vi "obj_DataLog Aggregate New Points.vi"(0 "method":T1, 9 "tag index in":i32) -> (10 "tag index out":i32)   [LabVIEW 2012]
doc: "This object aggregates the newly buffered points. This causes the points to be copied from the tag buffer to the aggregation buffer in a manner that is dependent on the selected logging algorithm and its parameterisation.\n\nThis object is called periodically by the aggregator plug-in. It is also called when a tag of the live database is being queried so as to move all available data over to the aggregation buffer for flush preceding the retrieval. This object is protected such that {aggregate} calls before {initialize} or after {cleanup} are inert."
uses:
  typedefs/t_DataLog Aggregate New Points Methods.ctl
  typedefs/clusters/t_DataLog Point.ctl
  typedefs/t_DataLog Tag Buffers Methods.ctl
  typedefs/t_DataLog Tag Info List Methods.ctl
  typedefs/t_DataLog Aggregation Buffer Methods.ctl
  subvis/private/glb_DataLog Runtime Parameterisation.vi
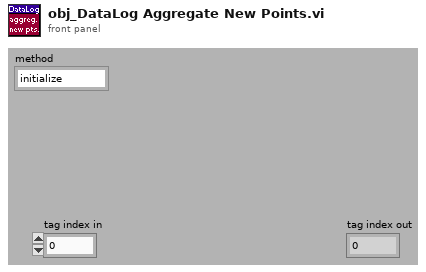
[diagram p1: front panel]
types:
  T1 = typedef "t_DataLog Aggregate New Points Methods.ctl" = enum16{"initialize", "aggregate", "cleanup"}
  T2 = typedef "t_DataLog Point.ctl" = cluster{"time":dbl, "value":dbl}
  T3 = typedef "t_DataLog Tag Buffers Methods.ctl" = enum16{"initialize", "inert", "write", "read", "read oldest", "read last", "cleanup"}
  T4 = typedef "t_DataLog Tag Info List Methods.ctl" = enum16{"initialize", "create", "create empty", "rename", "delete", "test tag", "get", "get by name", "get default", "get list", "get path", "get subsets", "set subsets", "set config", "set capacity", "#tags", "go live", "set unlocked", "set mirrored"}
  T5 = typedef "t_DataLog Aggregation Buffer Methods.ctl" = enum16{"initialize", "write", "write special", "flush", "flush next", "flush next if", "setup recovery", "update recovery", "verify recovery", "dummy flush ", "cleanup"}
  T6 = typedef "t_DataLog Tag Config.ctl" = cluster{"name":string, "unit":string, "temporal":T7, "value":T8, "index":i32, "capacity":i32, "is meta?":bool, "mincapacity":i32, "deadband":dbl, "limit delay":dbl, "format":T9, "precision":u8, "undefine":bool, "update":bool, "update period":u16, "expression":string, "description":string, "logging algorithm":T10, "logging parameters":dbl[]}
  T7 = typedef "t_DataLog Temporal Types.ctl" = enum16{"set&hold", "sample", "event"}
  T8 = typedef "t_DataLog Value Types.ctl" = enum16{"number", "string"}
  T9 = typedef "t_DataLog Numerical Format.ctl" = enum8{"fractional", "exponential", "engineering"}
  T10 = typedef "t_DataLog Logging Algorithms.ctl" = enum16{"nothing", "changes", "everything", "every Nth", "time threshold", "value threshold + prior", "t or v threshold", "t or v threshold + prior"}
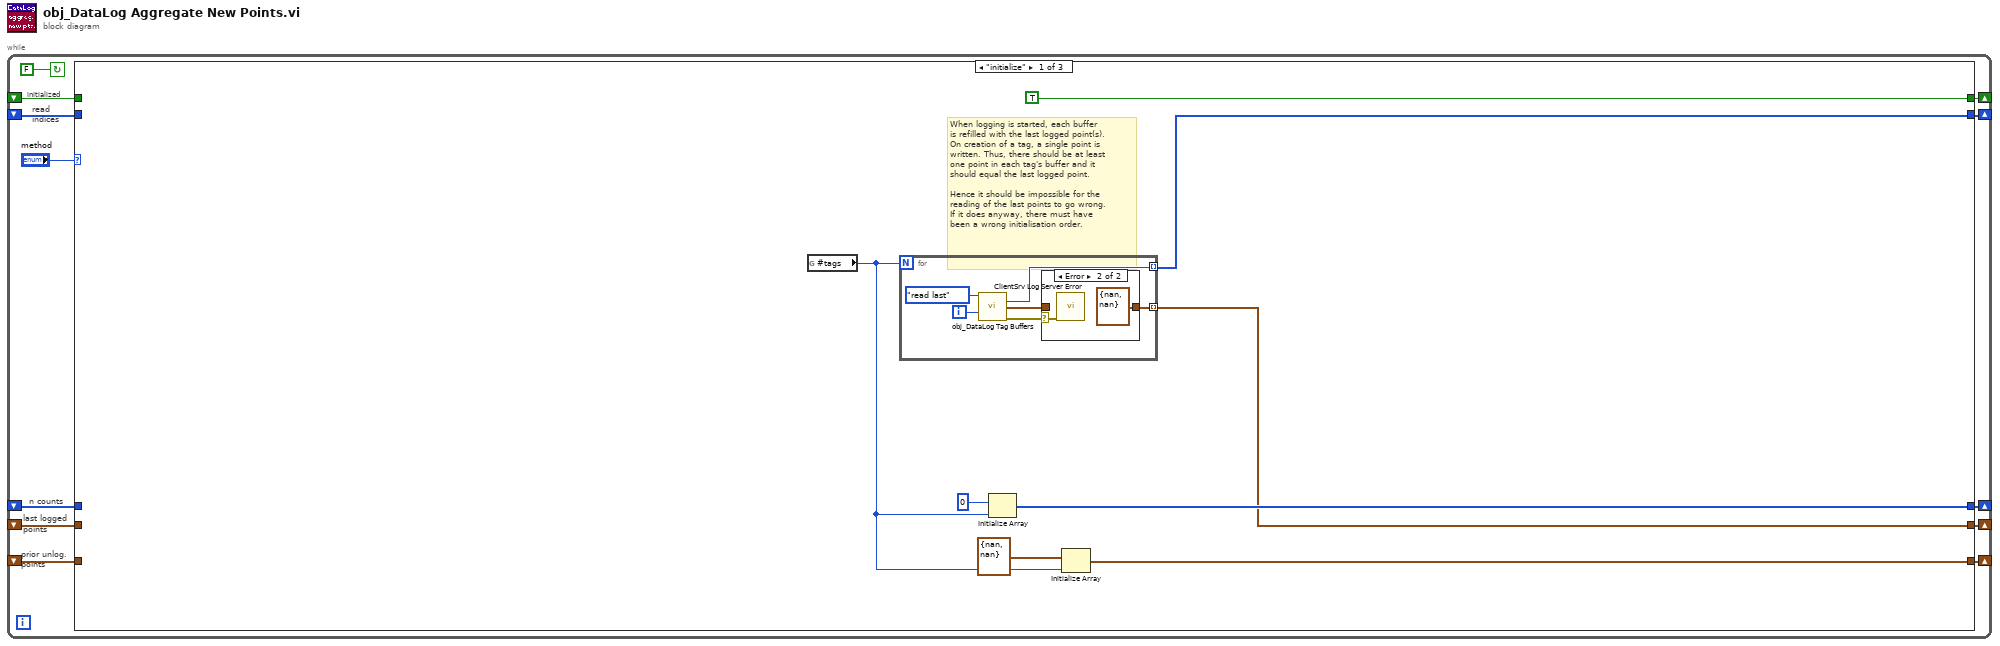
[diagram p0: block diagram]
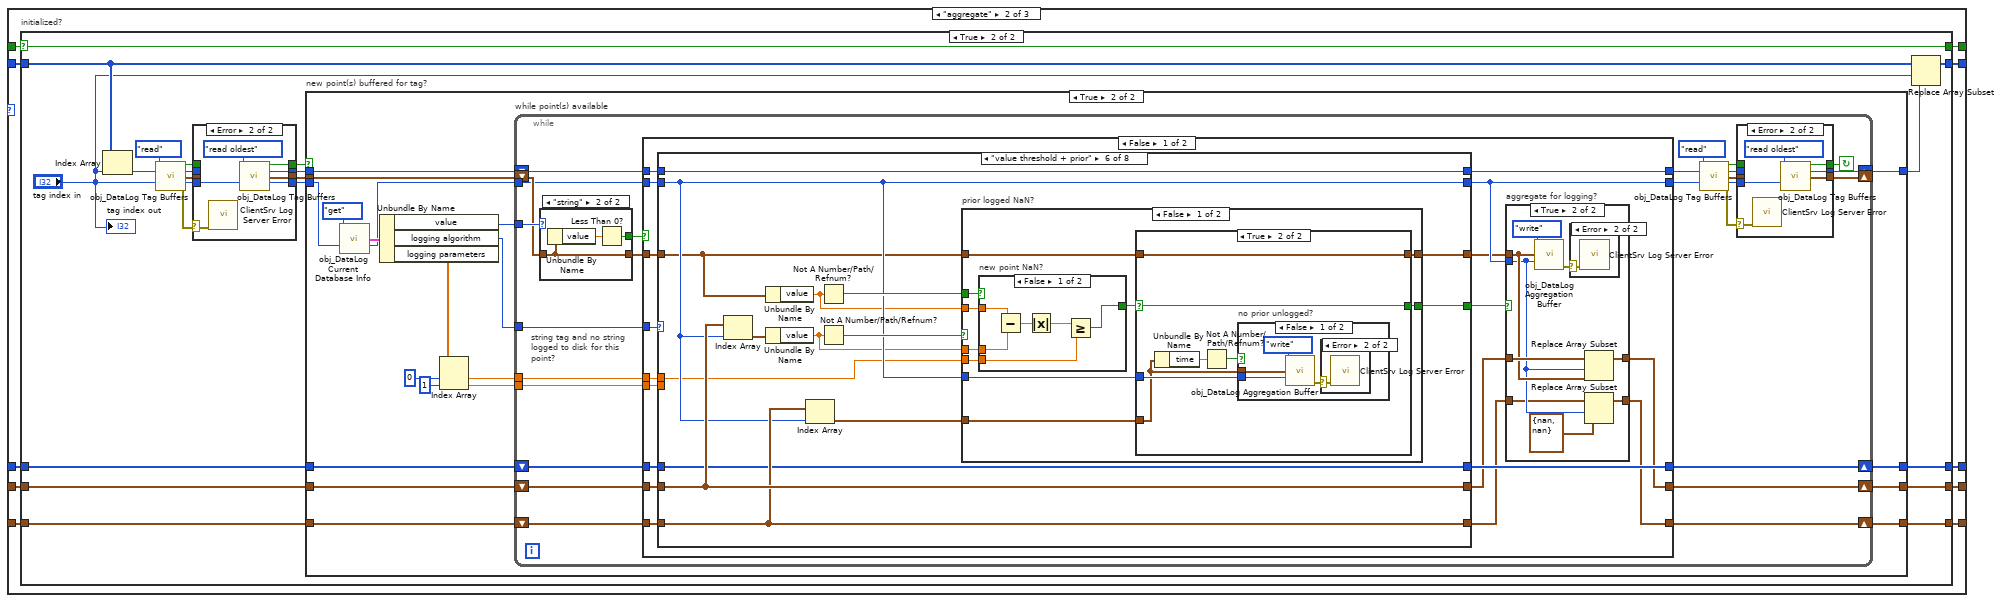
[diagram p3: hidden frame]
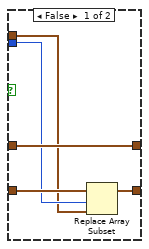
[diagram p8: hidden frame]
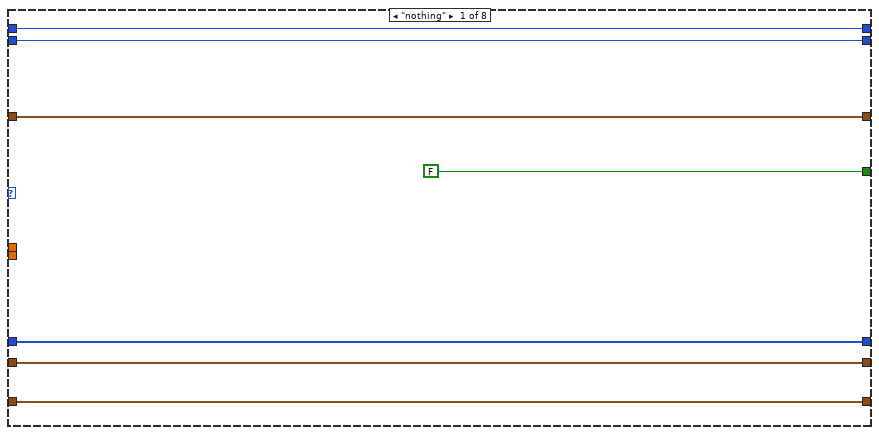
[diagram p10: hidden frame]
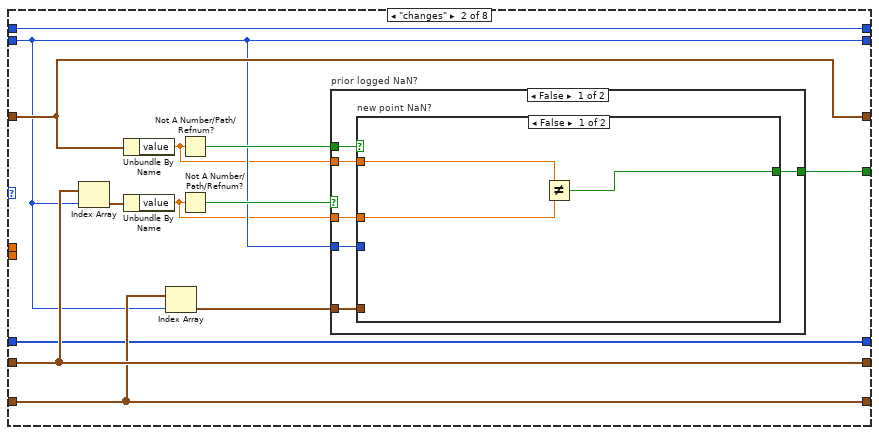
[diagram p11: hidden frame]
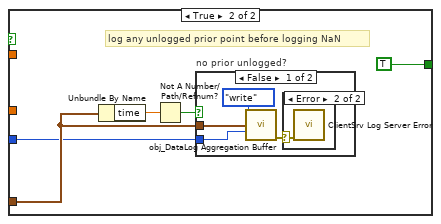
[diagram p12: hidden frame]
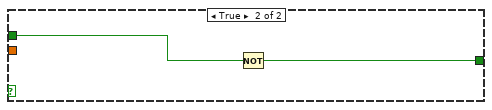
[diagram p15: hidden frame]
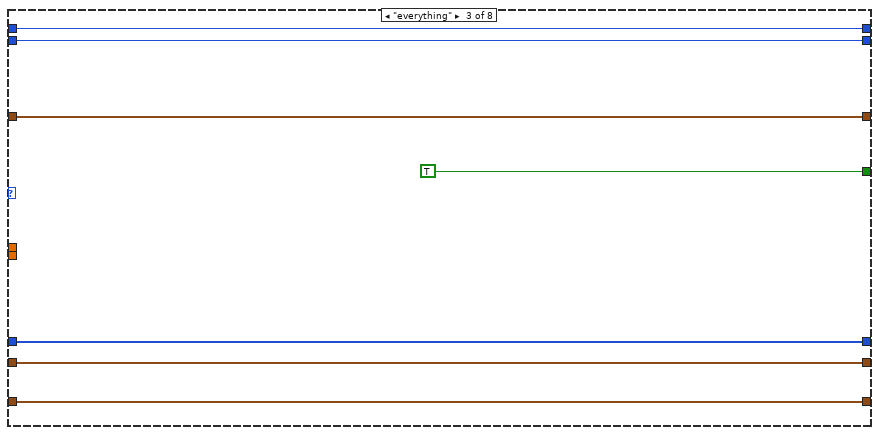
[diagram p16: hidden frame]
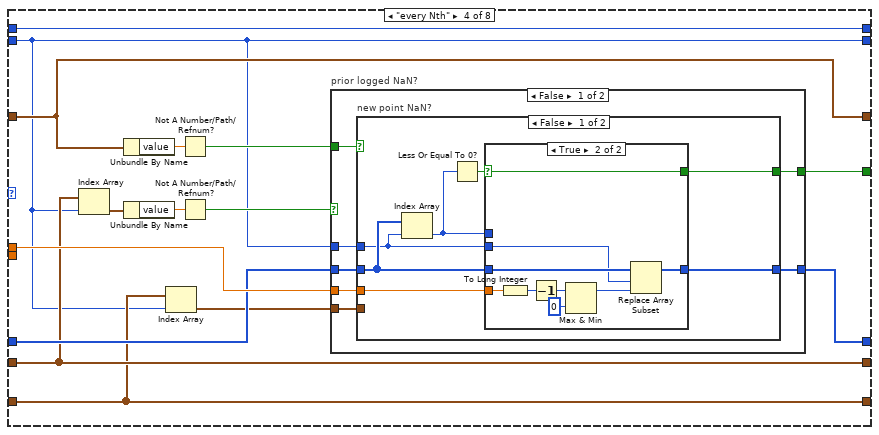
[diagram p17: hidden frame]
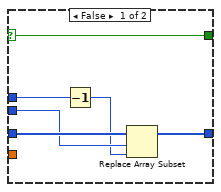
[diagram p18: hidden frame]
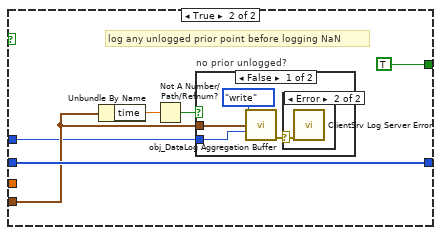
[diagram p19: hidden frame]
diagram:
  n1 = while {
    shift-right: [w9] -> _
    shift-left: _ -> [w10]
    shift-right: [w8] -> _
    shift-left: _ -> [w7]
    shift-right: [w6] -> _
    shift-left: _ -> [w5]
    shift-right: [w4] -> _
    shift-left: _ -> [w3]
    shift-right: [w2] -> _
    shift-left: _ -> [w1]
    stop <- FALSE continue-if-true
    # "prior unlog.\npoints"
    # "last logged\npoints"
    # "n counts"
    # "initialized"
    # "read\nindices"
    n2 = case shown="\"initialize\"" "method" {
      tunnel: w10 -> [_ w39 w520]
      tunnel: [w20 w38 w519] -> w9
      tunnel: [TRUE w36 FALSE] -> w8
      tunnel: w7 -> [_ w37 _]
      tunnel: [w17 w34 w515] -> w6
      tunnel: w5 -> [_ w35 w516]
      tunnel: [w13 w32 w512] -> w4
      tunnel: w3 -> [_ w33 w511]
      tunnel: [w15 w31 w508] -> w2
      tunnel: w1 -> [_ w30 w509]
      frame "initialize" {
        # "When logging is started, each buffer\nis refilled with the last logged point(s).\nOn creation of a tag, a single point is\nwritten. Thus, there should be at least\none point in each tag's buffer and it\nshould equal the last logged point.\n\nHence it should be impossible for the\nreading of the last points to go wrong.\nIf it does anyway, there must have\nbeen a wrong initialisation order."
        n3 = global read "glb_DataLog Runtime Parameterisation.vi" "#tags"() -> (w14:i32)
        n4 = for {
          N: w14 -> [_]
          tunnel: [w24] -> w20 mode=indexing
          tunnel: [w21] -> w13 mode=indexing
          i -> [w25]
          n5 = call "obj_DataLog Tag Buffers.vi"("method"=t_DataLog_Tag_Buffers_Methods."read last", "tag index"=w25) -> ("read index out"=w24:i32, "point out"=w22:T2, "error out"=w23:errorcluster)  [unwired: 9 in, 2 out]
          n6 = case shown="Error" w23 {
            selector: w23 -> [_ w29]
            tunnel: w22 -> [w27 _]
            tunnel: [w27 T2 {"time"=nan, "value"=nan} ("point")] -> w21
            frame No Error {
            }
            frame Error {
              n7 = call "ClientSrv Log Server Error.vi"("error (use message)"=w29) -> ()  [unwired: 15 in]
            }
          }
        }
        n8 = Initialize Array(0, w14) -> (w17:i32[])
        n9 = Initialize Array(T2 {"time"=nan, "value"=nan} ("point"), w14) -> (w15:T2[])
      }
      frame "aggregate" {
        n10 = case "initialized?" shown="True" w37 {
          selector: w37 -> [w44 w63]
          tunnel: w39 -> [w43 w66]
          tunnel: [w43 w65] -> w38
          tunnel: [w44 w63] -> w36
          tunnel: w35 -> [w42 w62]
          tunnel: [w42 w61] -> w34
          tunnel: [w41 w59] -> w32
          tunnel: w33 -> [w41 w60]
          tunnel: [w40 w58] -> w31
          tunnel: w30 -> [w40 w57]
          frame False {
            # "protects against on-query flush calls when aggregation is inactive"
          }
          frame True {
            n11 = Index Array(array=w66, index="tag index in") -> (element=w50:i32)
            n12 = call "obj_DataLog Tag Buffers.vi"("method"=t_DataLog_Tag_Buffers_Methods."read", "read index in"=w50, "tag index"="tag index in") -> ("available?"=w53:bool, "read index out"=w51:i32, "point out"=w55:T2, "tag index dup"=w54:i32, "error out"=w52:errorcluster)  [unwired: 8 in]
            n13 = case shown="Error" w52 {
              selector: w52 -> [_ w501]
              tunnel: w55 -> [w498 _]
              tunnel: w54 -> [w497 w503]
              tunnel: w53 -> [w499 _]
              tunnel: [w500 w506] -> w48
              tunnel: w51 -> [w500 _]
              tunnel: [w499 w505] -> w47
              tunnel: [w498 w504] -> w49
              tunnel: [w497 w502] -> w45
              frame No Error {
              }
              frame Error {
                n14 = call "ClientSrv Log Server Error.vi"("error (use message)"=w501) -> ()  [unwired: 15 in]
                n15 = call "obj_DataLog Tag Buffers.vi"("method"=t_DataLog_Tag_Buffers_Methods."read oldest", "tag index"=w503) -> ("available?"=w505:bool, "read index out"=w506:i32, "point out"=w504:T2, "tag index dup"=w502:i32)  [unwired: 9 in, 1 out]
              }
            }
            n16 = case "new point(s) buffered for tag?" shown="True" w47 {
              tunnel: [w70 w90] -> w64
              tunnel: w62 -> [w69 w89]
              tunnel: [w69 w88] -> w61
              tunnel: w60 -> [w68 w87]
              tunnel: [w68 w86] -> w59
              tunnel: [w67 w85] -> w58
              tunnel: w57 -> [w67 w84]
              tunnel: w49 -> [_ w83]
              tunnel: w48 -> [w70 w82]
              tunnel: w45 -> [_ w80]
              frame False {
              }
              frame True {
                n17 = call "obj_DataLog Current Database Info.vi"("method"=t_DataLog_Tag_Info_List_Methods."get", "tag index/change#"=w80) -> ("tag config out"=w79:T6, "dup tag index"=w71:i32)  [unwired: 7 in, 5 out]
                n18 = Unbundle By Name(w79) -> ("value"=w72:T8, "logging algorithm"=w75:T10, "logging parameters"=w76:dbl[])
                n19 = Index Array(array=w76, index #1=0 ("index"), index #2=1 ("index")) -> (element #1=w74:dbl, element #2=w73:dbl)
                n20 = while "while point(s) available" {
                  shift-right: [w96] -> w90
                  shift-left: w82 -> [w110]
                  shift-right: [w115] -> w88
                  shift-left: w89 -> [w116]
                  shift-right: [w113] -> w86
                  shift-left: w87 -> [w114]
                  shift-right: [w91] -> w85
                  shift-left: w84 -> [w92]
                  shift-right: [w95] -> _
                  shift-left: w83 -> [w105]
                  tunnel: w75 -> [w109]
                  tunnel: w74 -> [w108]
                  tunnel: w73 -> [w107]
                  tunnel: w72 -> [w106]
                  tunnel: w71 -> [w94]
                  stop <- w97 continue-if-true
                  n21 = case shown="\"string\"" w106 {
                    tunnel: w105 -> [w126 w127]
                    tunnel: [_ w128] -> w112
                    tunnel: [w126 w127] -> w111
                    frame "number" {
                    }
                    frame "string" {
                      n22 = Unbundle By Name(w127) -> ("value"=w129:dbl)
                      n23 = Less Than 0?(x=w129) -> (x < 0?=w128:bool)
                    }
                  }
                  n24 = case "string tag and no string logged to disk for this point?" shown="False" w112 {
                    tunnel: w110 -> [w147 w493]
                    tunnel: [w146 w493] -> w98
                    tunnel: w111 -> [w145 _]
                    tunnel: w109 -> [w144 _]
                    tunnel: w116 -> [w143 w496]
                    tunnel: [w142 w496] -> w115
                    tunnel: w114 -> [w141 w495]
                    tunnel: [w133 w495] -> w113
                    tunnel: w108 -> [w140 _]
                    tunnel: w107 -> [w139 _]
                    tunnel: w94 -> [w138 w494]
                    tunnel: [w136 w494] -> w93
                    tunnel: w92 -> [w137 w492]
                    tunnel: [w130 w492] -> w91
                    frame False {
                      n25 = case shown="\"value threshold + prior\"" w144 {
                        tunnel: w145 -> [w164 w176 w205 w214 w289 w324 w384 w435]
                        tunnel: w147 -> [w166 w182 w210 w223 w297 w337 w390 w441]
                        tunnel: [w166 w182 w210 w223 w297 w337 w390 w441] -> w146
                        tunnel: w143 -> [w169 w172 w209 w222 w283 w328 w378 w429]
                        tunnel: [w169 w172 w209 w225 w283 w328 w378 w429] -> w142
                        tunnel: w141 -> [w168 w180 w208 w218 w293 w335 w388 w439]
                        tunnel: [w168 w180 w208 w218 w293 w335 w388 w439] -> w135
                        tunnel: w140 -> [_ _ _ w224 w298 w325 w391 w442]
                        tunnel: w139 -> [_ _ _ _ _ _ w375 w426]
                        tunnel: w138 -> [w167 w174 w207 w212 w287 w330 w382 w433]
                        tunnel: [w167 w174 w207 w212 w287 w330 w382 w433] -> w136
                        tunnel: w137 -> [w165 w175 w206 w213 w288 w331 w383 w434]
                        tunnel: [w165 w175 w206 w213 w288 w331 w383 w434] -> w131
                        tunnel: [w164 w176 w205 w214 w289 w323 w384 w435] -> w134
                        tunnel: [FALSE w181 TRUE w221 w296 w336 w389 w440] -> w132
                        frame "nothing" {
                        }
                        frame "changes" {
                          n26 = Index Array(array=w180, index=w174) -> (element=w179:T2)
                          n27 = Unbundle By Name(w176) -> ("value"=w171:dbl)
                          n28 = Unbundle By Name(w179) -> ("value"=w170:dbl)
                          n29 = Index Array(array=w175, index=w174) -> (element=w173:T2)
                          n30 = Not A Number/Path/Refnum?(number/path/refnum=w171) -> (NaN/Path/Refnum?=w178:bool)
                          n31 = Not A Number/Path/Refnum?(number/path/refnum=w170) -> (NaN/Path/Refnum?=w177:bool)
                          n32 = case "prior logged NaN?" shown="False" w177 {
                            tunnel: [w188 w203] -> w181
                            tunnel: w174 -> [w187 _]
                            tunnel: w178 -> [w186 w202]
                            tunnel: w173 -> [w185 _]
                            tunnel: w170 -> [w184 _]
                            tunnel: w171 -> [w183 _]
                            frame False {
                              n33 = case "new point NaN?" shown="False" w186 {
                                tunnel: [w189 TRUE] -> w188
                                tunnel: w187 -> [_ w192]
                                tunnel: w185 -> [_ w193]
                                tunnel: w184 -> [w190 _]
                                tunnel: w183 -> [w191 _]
                                frame False {
                                n34 = Not Equal?(x=w191, y=w190) -> (x != y?=w189:bool)
                                }
                                frame True {
                                # "log any unlogged prior point before logging NaN"
                                n35 = Unbundle By Name(w193) -> ("time"=w195:dbl)
                                n36 = Not A Number/Path/Refnum?(number/path/refnum=w195) -> (NaN/Path/Refnum?=w194:bool)
                                n37 = case "no prior unlogged?" shown="False" w194 {
                                tunnel: w193 -> [w198 _]
                                tunnel: w192 -> [w197 _]
                                frame False {
                                n38 = call "obj_DataLog Aggregation Buffer.vi"("method"=t_DataLog_Aggregation_Buffer_Methods."write", "point"=w198, "tag index"=w197) -> ("error out"=w200:errorcluster)  [unwired: 11 in, 1 out]
                                n39 = case shown="Error" w200 {
                                selector: w200 -> [_ w201]
                                frame No Error {
                                }
                                frame Error {
                                n40 = call "ClientSrv Log Server Error.vi"("error (use message)"=w201) -> ()  [unwired: 15 in]
                                }
                                }
                                }
                                frame True {
                                }
                                }
                                }
                              }
                            }
                            frame True {
                              n41 = Not(x=w202) -> (.not. x?=w203:bool)
                            }
                          }
                        }
                        frame "everything" {
                        }
                        frame "every Nth" {
                          n42 = Index Array(array=w218, index=w212) -> (element=w217:T2)
                          n43 = Unbundle By Name(w214) -> ("value"=w220:dbl)
                          n44 = Unbundle By Name(w217) -> ("value"=w219:dbl)
                          n45 = Index Array(array=w213, index=w212) -> (element=w211:T2)
                          n46 = Not A Number/Path/Refnum?(number/path/refnum=w220) -> (NaN/Path/Refnum?=w216:bool)
                          n47 = Not A Number/Path/Refnum?(number/path/refnum=w219) -> (NaN/Path/Refnum?=w215:bool)
                          n48 = case "prior logged NaN?" shown="False" w215 {
                            tunnel: [w232 w271] -> w225
                            tunnel: w224 -> [w231 w270]
                            tunnel: w222 -> [w230 w269]
                            tunnel: [w229 w268] -> w221
                            tunnel: w212 -> [w228 w267]
                            tunnel: w216 -> [w227 w266]
                            tunnel: w211 -> [w226 _]
                            frame False {
                              n49 = case "new point NaN?" shown="False" w227 {
                                tunnel: [w239 w259] -> w232
                                tunnel: w231 -> [w238 _]
                                tunnel: w230 -> [w236 w259]
                                tunnel: [w237 TRUE] -> w229
                                tunnel: w228 -> [w235 w255]
                                tunnel: w226 -> [_ w256]
                                frame False {
                                n50 = Index Array(array=w236, index=w235) -> (element=w233:i32)
                                n51 = Less Or Equal To 0?(x=w233) -> (x <= 0?=w234:bool)
                                n52 = case shown="True" w234 {
                                selector: w234 -> [w241 w246]
                                tunnel: w235 -> [w243 w252]
                                tunnel: w236 -> [w245 w254]
                                tunnel: [w244 w251] -> w239
                                tunnel: w238 -> [_ w247]
                                tunnel: [w241 w246] -> w237
                                tunnel: w233 -> [w240 _]
                                frame False {
                                n53 = Decrement(x=w240) -> (x-1=w242:i32)
                                n54 = Replace Array Subset(array=w245, new element=w242, index=w243) -> (w244:i32[])
                                }
                                frame True {
                                n55 = To Long Integer(number=w247) -> (32bit integer=w253:i32)
                                n56 = Decrement(x=w253) -> (x-1=w250:i32)
                                n57 = Max & Min(x=w250, y=0) -> (max(x,y)=w249:i32)  [unwired: 1 out]
                                n58 = Replace Array Subset(array=w254, new element=w249, index=w252) -> (w251:i32[])
                                }
                                }
                                }
                                frame True {
                                # "log any unlogged prior point before logging NaN"
                                n59 = Unbundle By Name(w256) -> ("time"=w258:dbl)
                                n60 = Not A Number/Path/Refnum?(number/path/refnum=w258) -> (NaN/Path/Refnum?=w257:bool)
                                n61 = case "no prior unlogged?" shown="False" w257 {
                                tunnel: w256 -> [w262 _]
                                tunnel: w255 -> [w261 _]
                                frame False {
                                n62 = call "obj_DataLog Aggregation Buffer.vi"("method"=t_DataLog_Aggregation_Buffer_Methods."write", "point"=w262, "tag index"=w261) -> ("error out"=w264:errorcluster)  [unwired: 11 in, 1 out]
                                n63 = case shown="Error" w264 {
                                selector: w264 -> [_ w265]
                                frame No Error {
                                }
                                frame Error {
                                n64 = call "ClientSrv Log Server Error.vi"("error (use message)"=w265) -> ()  [unwired: 15 in]
                                }
                                }
                                }
                                frame True {
                                }
                                }
                                }
                              }
                            }
                            frame True {
                              n65 = case "new NaN?" shown="False" w266 {
                                tunnel: [w274 w282] -> w271
                                tunnel: w270 -> [w275 _]
                                tunnel: w269 -> [w279 w282]
                                tunnel: [TRUE FALSE] -> w268
                                tunnel: w267 -> [w273 _]
                                frame False {
                                n66 = To Long Integer(number=w275) -> (32bit integer=w278:i32)
                                n67 = Decrement(x=w278) -> (x-1=w277:i32)
                                n68 = Max & Min(x=w277, y=0) -> (max(x,y)=w272:i32)  [unwired: 1 out]
                                n69 = Replace Array Subset(array=w279, new element=w272, index=w273) -> (w274:i32[])
                                }
                                frame True {
                                }
                              }
                            }
                          }
                        }
                        frame "time threshold" {
                          n70 = Index Array(array=w293, index=w287) -> (element=w292:T2)
                          n71 = Unbundle By Name(w289) -> ("value"=w295:dbl, "time"=w284:dbl)
                          n72 = Unbundle By Name(w292) -> ("value"=w294:dbl, "time"=w285:dbl)
                          n73 = Index Array(array=w288, index=w287) -> (element=w286:T2)
                          n74 = Not A Number/Path/Refnum?(number/path/refnum=w295) -> (NaN/Path/Refnum?=w291:bool)
                          n75 = Not A Number/Path/Refnum?(number/path/refnum=w294) -> (NaN/Path/Refnum?=w290:bool)
                          n76 = case "prior logged NaN?" shown="False" w290 {
                            tunnel: w298 -> [w305 _]
                            tunnel: [w304 w322] -> w296
                            tunnel: w287 -> [w303 _]
                            tunnel: w291 -> [w302 w321]
                            tunnel: w286 -> [w301 _]
                            tunnel: w285 -> [w300 _]
                            tunnel: w284 -> [w299 _]
                            frame False {
                              n77 = case "new point NaN?" shown="False" w302 {
                                tunnel: w305 -> [w307 _]
                                tunnel: [w306 TRUE] -> w304
                                tunnel: w303 -> [_ w311]
                                tunnel: w301 -> [_ w312]
                                tunnel: w300 -> [w309 _]
                                tunnel: w299 -> [w310 _]
                                frame False {
                                n78 = Subtract(x=w310, y=w309) -> (x-y=w308:dbl)
                                n79 = Greater Or Equal?(x=w308, y=w307) -> (x >= y?=w306:bool)
                                }
                                frame True {
                                # "log any unlogged prior point before logging NaN"
                                n80 = Unbundle By Name(w312) -> ("time"=w314:dbl)
                                n81 = Not A Number/Path/Refnum?(number/path/refnum=w314) -> (NaN/Path/Refnum?=w313:bool)
                                n82 = case "no prior unlogged?" shown="False" w313 {
                                tunnel: w312 -> [w317 _]
                                tunnel: w311 -> [w316 _]
                                frame False {
                                n83 = call "obj_DataLog Aggregation Buffer.vi"("method"=t_DataLog_Aggregation_Buffer_Methods."write", "point"=w317, "tag index"=w316) -> ("error out"=w319:errorcluster)  [unwired: 11 in, 1 out]
                                n84 = case shown="Error" w319 {
                                selector: w319 -> [_ w320]
                                frame No Error {
                                }
                                frame Error {
                                n85 = call "ClientSrv Log Server Error.vi"("error (use message)"=w320) -> ()  [unwired: 15 in]
                                }
                                }
                                }
                                frame True {
                                }
                                }
                                }
                              }
                            }
                            frame True {
                              n86 = Not(x=w321) -> (.not. x?=w322:bool)
                            }
                          }
                        }
                        frame "value threshold + prior" {
                          n87 = Index Array(array=w335, index=w330) -> (element=w334:T2)
                          n88 = Unbundle By Name(w324) -> ("value"=w327:dbl)
                          n89 = Unbundle By Name(w334) -> ("value"=w326:dbl)
                          n90 = Index Array(array=w331, index=w330) -> (element=w329:T2)
                          n91 = Not A Number/Path/Refnum?(number/path/refnum=w327) -> (NaN/Path/Refnum?=w333:bool)
                          n92 = Not A Number/Path/Refnum?(number/path/refnum=w326) -> (NaN/Path/Refnum?=w332:bool)
                          n93 = case "prior logged NaN?" shown="False" w332 {
                            tunnel: [w340 w374] -> w336
                            tunnel: w330 -> [w343 _]
                            tunnel: w333 -> [w347 w373]
                            tunnel: w329 -> [w342 _]
                            tunnel: w326 -> [w346 _]
                            tunnel: w327 -> [w345 _]
                            tunnel: w325 -> [w344 _]
                            tunnel: w324 -> [w339 w372]
                            tunnel: [w338 w372] -> w323
                            frame False {
                              n94 = case "new point NaN?" shown="False" w347 {
                                selector: w347 -> [_ w371]
                                tunnel: [w365 w371] -> w341
                                tunnel: w346 -> [w368 _]
                                tunnel: w345 -> [w369 _]
                                tunnel: w344 -> [w366 _]
                                frame False {
                                n95 = Subtract(x=w369, y=w368) -> (x-y=w370:dbl)
                                n96 = Absolute Value(x=w370) -> (abs(x)=w367:dbl)
                                n97 = Greater Or Equal?(x=w367, y=w366) -> (x >= y?=w365:bool)
                                }
                                frame True {
                                }
                              }
                              n98 = case shown="True" w341 {
                                selector: w341 -> [w352 w355]
                                tunnel: w343 -> [w348 w357]
                                tunnel: w342 -> [_ w356]
                                tunnel: [w352 w355] -> w340
                                tunnel: w339 -> [w349 w354]
                                tunnel: [w349 w354] -> w338
                                frame False {
                                # "ensure that no large timerange will be uninterpolatable when the system crashes which might otherwise happen when the signal value remains nearly constant for a long time"
                                n99 = call "obj_DataLog Aggregation Buffer.vi"("method"=t_DataLog_Aggregation_Buffer_Methods."write special", "point"=w349, "tag index"=w348) -> ("error out"=w350:errorcluster)  [unwired: 11 in, 1 out]
                                n100 = case shown="Error" w350 {
                                selector: w350 -> [_ w353]
                                frame No Error {
                                }
                                frame Error {
                                n101 = call "ClientSrv Log Server Error.vi"("error (use message)"=w353) -> ()  [unwired: 15 in]
                                }
                                }
                                }
                                frame True {
                                n102 = Unbundle By Name(w356) -> ("time"=w359:dbl)
                                n103 = Not A Number/Path/Refnum?(number/path/refnum=w359) -> (NaN/Path/Refnum?=w358:bool)
                                n104 = case "no prior unlogged?" shown="False" w358 {
                                tunnel: w356 -> [w361 _]
                                tunnel: w357 -> [w360 _]
                                frame False {
                                n105 = call "obj_DataLog Aggregation Buffer.vi"("method"=t_DataLog_Aggregation_Buffer_Methods."write", "point"=w361, "tag index"=w360) -> ("error out"=w363:errorcluster)  [unwired: 11 in, 1 out]
                                n106 = case shown="Error" w363 {
                                selector: w363 -> [_ w364]
                                frame No Error {
                                }
                                frame Error {
                                n107 = call "ClientSrv Log Server Error.vi"("error (use message)"=w364) -> ()  [unwired: 15 in]
                                }
                                }
                                }
                                frame True {
                                }
                                }
                                }
                              }
                            }
                            frame True {
                              n108 = Not(x=w373) -> (.not. x?=w374:bool)
                            }
                          }
                        }
                        frame "t or v threshold" {
                          n109 = Index Array(array=w388, index=w382) -> (element=w387:T2)
                          n110 = Unbundle By Name(w384) -> ("value"=w376:dbl, "time"=w379:dbl)
                          n111 = Unbundle By Name(w387) -> ("value"=w377:dbl, "time"=w380:dbl)
                          n112 = Index Array(array=w383, index=w382) -> (element=w381:T2)
                          n113 = Not A Number/Path/Refnum?(number/path/refnum=w376) -> (NaN/Path/Refnum?=w386:bool)
                          n114 = Not A Number/Path/Refnum?(number/path/refnum=w377) -> (NaN/Path/Refnum?=w385:bool)
                          n115 = case "prior logged NaN?" shown="False" w385 {
                            tunnel: w391 -> [w401 _]
                            tunnel: [w400 w425] -> w389
                            tunnel: w382 -> [w399 _]
                            tunnel: w386 -> [w398 w424]
                            tunnel: w381 -> [w397 _]
                            tunnel: w380 -> [w396 _]
                            tunnel: w379 -> [w395 _]
                            tunnel: w377 -> [w394 _]
                            tunnel: w376 -> [w393 _]
                            tunnel: w375 -> [w392 _]
                            frame False {
                              n116 = case "new point NaN?" shown="False" w398 {
                                tunnel: w401 -> [w410 _]
                                tunnel: [w402 TRUE] -> w400
                                tunnel: w399 -> [_ w414]
                                tunnel: w397 -> [_ w415]
                                tunnel: w396 -> [w412 _]
                                tunnel: w395 -> [w413 _]
                                tunnel: w394 -> [w408 _]
                                tunnel: w393 -> [w409 _]
                                tunnel: w392 -> [w405 _]
                                frame False {
                                n117 = Subtract(x=w409, y=w408) -> (x-y=w407:dbl)
                                n118 = Absolute Value(x=w407) -> (abs(x)=w406:dbl)
                                n119 = Greater Or Equal?(x=w406, y=w405) -> (x >= y?=w404:bool)
                                n120 = Subtract(x=w413, y=w412) -> (x-y=w411:dbl)
                                n121 = Greater Or Equal?(x=w411, y=w410) -> (x >= y?=w403:bool)
                                n122 = Or(x=w404, y=w403) -> (x .or. y?=w402:bool)
                                }
                                frame True {
                                # "log any unlogged prior point before logging NaN"
                                n123 = Unbundle By Name(w415) -> ("time"=w417:dbl)
                                n124 = Not A Number/Path/Refnum?(number/path/refnum=w417) -> (NaN/Path/Refnum?=w416:bool)
                                n125 = case "no prior unlogged?" shown="False" w416 {
                                tunnel: w415 -> [w420 _]
                                tunnel: w414 -> [w419 _]
                                frame False {
                                n126 = call "obj_DataLog Aggregation Buffer.vi"("method"=t_DataLog_Aggregation_Buffer_Methods."write", "point"=w420, "tag index"=w419) -> ("error out"=w422:errorcluster)  [unwired: 11 in, 1 out]
                                n127 = case shown="Error" w422 {
                                selector: w422 -> [_ w423]
                                frame No Error {
                                }
                                frame Error {
                                n128 = call "ClientSrv Log Server Error.vi"("error (use message)"=w423) -> ()  [unwired: 15 in]
                                }
                                }
                                }
                                frame True {
                                }
                                }
                                }
                              }
                            }
                            frame True {
                              n129 = Not(x=w424) -> (.not. x?=w425:bool)
                            }
                          }
                        }
                        frame "t or v threshold + prior" {
                          n130 = Index Array(array=w439, index=w433) -> (element=w438:T2)
                          n131 = Unbundle By Name(w435) -> ("value"=w427:dbl, "time"=w430:dbl)
                          n132 = Unbundle By Name(w438) -> ("value"=w428:dbl, "time"=w431:dbl)
                          n133 = Index Array(array=w434, index=w433) -> (element=w432:T2)
                          n134 = Not A Number/Path/Refnum?(number/path/refnum=w427) -> (NaN/Path/Refnum?=w437:bool)
                          n135 = Not A Number/Path/Refnum?(number/path/refnum=w428) -> (NaN/Path/Refnum?=w436:bool)
                          n136 = case "prior logged NaN?" shown="False" w436 {
                            tunnel: w442 -> [w452 _]
                            tunnel: [w451 w491] -> w440
                            tunnel: w433 -> [w450 _]
                            tunnel: w437 -> [w449 w490]
                            tunnel: w432 -> [w448 _]
                            tunnel: w431 -> [w447 _]
                            tunnel: w430 -> [w446 _]
                            tunnel: w428 -> [w445 _]
                            tunnel: w427 -> [w444 _]
                            tunnel: w426 -> [w443 _]
                            frame False {
                              n137 = case "new point NaN?" shown="False" w449 {
                                tunnel: w452 -> [w453 _]
                                tunnel: [w457 TRUE] -> w451
                                tunnel: w450 -> [w459 w480]
                                tunnel: w448 -> [w458 w481]
                                tunnel: w447 -> [w454 _]
                                tunnel: w446 -> [w455 _]
                                tunnel: w445 -> [w463 _]
                                tunnel: w444 -> [w464 _]
                                tunnel: w443 -> [w460 _]
                                frame False {
                                n138 = Subtract(x=w464, y=w463) -> (x-y=w462:dbl)
                                n139 = Absolute Value(x=w462) -> (abs(x)=w461:dbl)
                                n140 = Greater Or Equal?(x=w461, y=w460) -> (x >= y?=w456:bool)
                                n141 = case shown="True" w456 {
                                selector: w456 -> [_ w470]
                                tunnel: w459 -> [_ w472]
                                tunnel: w458 -> [_ w471]
                                tunnel: [w465 w470] -> w457
                                tunnel: w455 -> [w468 _]
                                tunnel: w454 -> [w467 _]
                                tunnel: w453 -> [w466 _]
                                frame False {
                                n142 = Subtract(x=w468, y=w467) -> (x-y=w469:dbl)
                                n143 = Greater Or Equal?(x=w469, y=w466) -> (x >= y?=w465:bool)
                                }
                                frame True {
                                n144 = Unbundle By Name(w471) -> ("time"=w474:dbl)
                                n145 = Not A Number/Path/Refnum?(number/path/refnum=w474) -> (NaN/Path/Refnum?=w473:bool)
                                n146 = case "no prior unlogged?" shown="False" w473 {
                                tunnel: w471 -> [w476 _]
                                tunnel: w472 -> [w475 _]
                                frame False {
                                n147 = call "obj_DataLog Aggregation Buffer.vi"("method"=t_DataLog_Aggregation_Buffer_Methods."write", "point"=w476, "tag index"=w475) -> ("error out"=w478:errorcluster)  [unwired: 11 in, 1 out]
                                n148 = case shown="Error" w478 {
                                selector: w478 -> [_ w479]
                                frame No Error {
                                }
                                frame Error {
                                n149 = call "ClientSrv Log Server Error.vi"("error (use message)"=w479) -> ()  [unwired: 15 in]
                                }
                                }
                                }
                                frame True {
                                }
                                }
                                }
                                }
                                }
                                frame True {
                                # "log any unlogged prior point before logging NaN"
                                n150 = Unbundle By Name(w481) -> ("time"=w483:dbl)
                                n151 = Not A Number/Path/Refnum?(number/path/refnum=w483) -> (NaN/Path/Refnum?=w482:bool)
                                n152 = case "no prior unlogged?" shown="False" w482 {
                                tunnel: w481 -> [w486 _]
                                tunnel: w480 -> [w485 _]
                                frame False {
                                n153 = call "obj_DataLog Aggregation Buffer.vi"("method"=t_DataLog_Aggregation_Buffer_Methods."write", "point"=w486, "tag index"=w485) -> ("error out"=w488:errorcluster)  [unwired: 11 in, 1 out]
                                n154 = case shown="Error" w488 {
                                selector: w488 -> [_ w489]
                                frame No Error {
                                }
                                frame Error {
                                n155 = call "ClientSrv Log Server Error.vi"("error (use message)"=w489) -> ()  [unwired: 15 in]
                                }
                                }
                                }
                                frame True {
                                }
                                }
                                }
                              }
                            }
                            frame True {
                              n156 = Not(x=w490) -> (.not. x?=w491:bool)
                            }
                          }
                        }
                      }
                      n157 = case "aggregate for logging?" shown="True" w132 {
                        tunnel: w136 -> [w149 w156]
                        tunnel: w135 -> [w152 w159]
                        tunnel: w134 -> [w148 w157]
                        tunnel: [w152 w158] -> w133
                        tunnel: w131 -> [w151 w155]
                        tunnel: [w150 w154] -> w130
                        frame False {
                          n158 = Replace Array Subset(array=w151, new element=w148, index=w149) -> (w150:T2[])
                        }
                        frame True {
                          n159 = call "obj_DataLog Aggregation Buffer.vi"("method"=t_DataLog_Aggregation_Buffer_Methods."write", "point"=w157, "tag index"=w156) -> ("error out"=w161:errorcluster)  [unwired: 11 in, 1 out]
                          n160 = case shown="Error" w161 {
                            selector: w161 -> [_ w162]
                            frame No Error {
                            }
                            frame Error {
                              n161 = call "ClientSrv Log Server Error.vi"("error (use message)"=w162) -> ()  [unwired: 15 in]
                            }
                          }
                          n162 = Replace Array Subset(array=w159, new element=w157, index=w156) -> (w158:T2[])
                          n163 = Replace Array Subset(array=w155, new element=T2 {"time"=nan, "value"=nan} ("point"), index=w156) -> (w154:T2[])
                        }
                      }
                    }
                    frame True {
                    }
                  }
                  n164 = call "obj_DataLog Tag Buffers.vi"("method"=t_DataLog_Tag_Buffers_Methods."read", "read index in"=w98, "tag index"=w93) -> ("available?"=w101:bool, "read index out"=w99:i32, "point out"=w103:T2, "tag index dup"=w102:i32, "error out"=w100:errorcluster)  [unwired: 8 in]
                  n165 = case shown="Error" w100 {
                    selector: w100 -> [_ w120]
                    tunnel: w103 -> [w117 _]
                    tunnel: w102 -> [_ w121]
                    tunnel: w101 -> [w118 _]
                    tunnel: [w119 w124] -> w96
                    tunnel: w99 -> [w119 _]
                    tunnel: [w118 w123] -> w97
                    tunnel: [w117 w122] -> w95
                    frame No Error {
                    }
                    frame Error {
                      n166 = call "ClientSrv Log Server Error.vi"("error (use message)"=w120) -> ()  [unwired: 15 in]
                      n167 = call "obj_DataLog Tag Buffers.vi"("method"=t_DataLog_Tag_Buffers_Methods."read oldest", "tag index"=w121) -> ("available?"=w123:bool, "read index out"=w124:i32, "point out"=w122:T2)  [unwired: 9 in, 2 out]
                    }
                  }
                }
              }
            }
            n168 = Replace Array Subset(array=w66, new element=w64, index="tag index in") -> (w65:i32[])
            "tag index out" <- "tag index in"
          }
        }
      }
      frame "cleanup" {
        n169 = Reshape Array(w516, 0 ("dimension size")) -> (w515:i32[])
        n170 = Reshape Array(w520, 0 ("dimension size")) -> (w519:i32[])
        n171 = Reshape Array(w511, 0 ("dimension size")) -> (w512:T2[])
        n172 = Reshape Array(w509, 0 ("dimension size")) -> (w508:T2[])
      }
    }
  }
